vi "SubVI_Gas Mark #.vi"(7 "Image Register Name":string="untitled", 8 "Error in":errorcluster, 9 "Divider":sgl format="%.2f", 10 "Kernel Size":i32=3 min=3 max=201 step=2, 11 "Image Src In":T1) -> (0 "Error out":errorcluster, 2 "Image Dst Out":T1, 3 "Image Src Out":T1)   [LabVIEW 2013]
uses:
  <vilib>/vision/Image Controls.llb/IMAQ Image.ctl
  <vilib>/vision/NI_Vision_Development_Module.lvlib
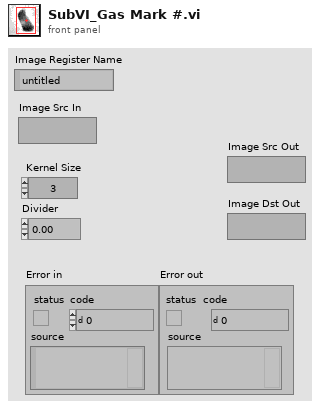
[diagram p1: front panel]
types:
  T1 = typedef "IMAQ Image.ctl" = refnum<image>
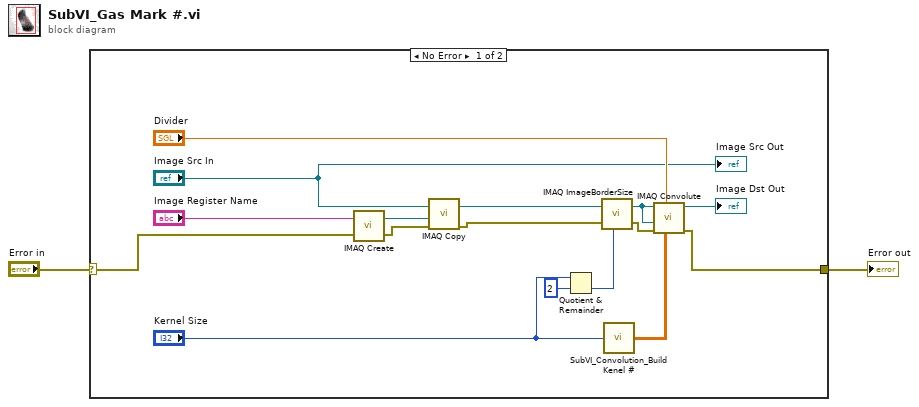
[diagram p0: block diagram]
diagram:
  n1 = case shown="No Error" "Error in" {
    selector: "Error in" -> [w7 w19]
    tunnel: [w3 w19] -> w1
    frame No Error {
      n2 = call "IMAQ Create"("Image Name"="Image Register Name", "error in (no error)"=w7) -> ("New Image"=w11:T1, "error out"=w6:errorcluster)  [unwired: 3 in]
      n3 = call "IMAQ Copy"("error in (no error)"=w6, "Image Dst"=w11, "Image Src"="Image Src In") -> ("error out"=w5:errorcluster, "Image Dst Out"=w10:T1)  [unwired: 3 in]
      n4 = Quotient & Remainder(x="Kernel Size", y=2) -> (floor(x/y)=w13:i32)  [unwired: 1 out]
      n5 = call "IMAQ ImageBorderSize"("Image"=w10, "Image border size in"=w13, "error in (no error)"=w5) -> ("Image Out"=w9:T1, "error out"=w4:errorcluster)  [unwired: 1 in, 1 out]
      n6 = call "SubVI_Convolution_Build Kenel #.vi"("Kernel Size"="Kernel Size") -> ("Kernel"=w18:sgl[][])
      n7 = call "IMAQ Convolute"("Kernel"=w18, "Divider (kernel sum)"="Divider", "error in (no error)"=w4, "Image Dst"=w9, "Image Src"=w9) -> ("error out"=w3:errorcluster, "Image Dst Out"=→"Image Dst Out":T1)  [unwired: 5 in]
      "Image Src Out" <- "Image Src In"
    }
    frame Error {
    }
  }
  "Error out" <- w1
